vi "End Run.vi"(8 "abort":bool, 11 "RTTarget in":refnum<class "RTTarget.lvclass">) -> (3 "RTTarget out":refnum<class "RTTarget.lvclass">)   [LabVIEW 2020, in "NI_TargetHelper.lvlib" / "RTTarget.lvclass"]
uses:
  <vilib>/TargetSupport/NI_TargetHelper/RTTarget/RTTarget.lvclass
  <vilib>/TargetSupport/NI_TargetHelper/RTTarget/RTTarget.lvclass/RTTarget.ctl
  <vilib>/TargetSupport/NI_TargetHelper/Run Target VI.ctl
  <vilib>/TargetSupport/NI_TargetHelper/NI_TargetHelper.lvlib
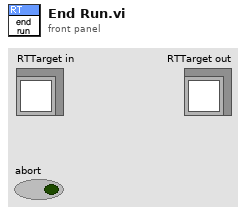
[diagram p1: front panel]
types:
  T1 = typedef "NI_TargetHelper.lvlib/Run Target VI.ctl" = refnum<vi>
  T2 = typedef "NI_TargetHelper.lvlib/Instance VIref.ctl" = refnum<vi>
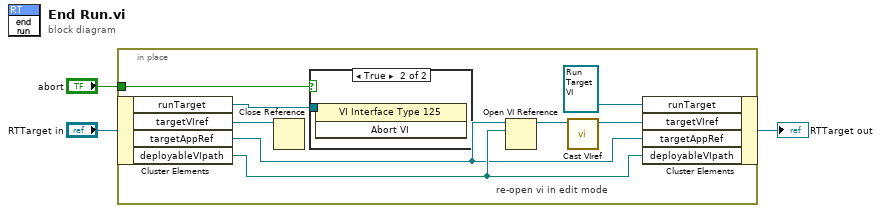
[diagram p0: block diagram]
diagram:
  n1 = in-place {
    in-place-border: "abort" -> [w10]
    # "re-open vi in edit mode"
    n2 = in-place-cluster #1("RTTarget in") -> ("runTarget"=w11:T1, "targetVIref"=w8:T2, "targetAppRef"=w4:refnum<vi>, "deployableVIpath"=w6:path)
    n3 = Close Reference(reference=w8) -> ()  [unwired: 1 in, 1 out]
    n4 = case shown="True" w10 {
      tunnel: w11 -> [_ w12]
      frame False {
      }
      frame True {
        n5 = invoke class="VI Interface Type 125" method="Abort VI"(reference=w12) -> ()  [unwired: 2 in, 3 out]
      }
    }
    n6 = Open VI Reference(application reference (local)=w4, vi path=w6) -> (vi reference=w7:refnum<vi>)  [unwired: 4 in, 1 out]
    n7 = call <vilib>:"Cast VIref.vi"("VI Refnum"=w7) -> ("instVIref"=w5:T2)  [unwired: 10 in]
    n8 = in-place-cluster #1("runTarget"=T1 refnum, "targetVIref"=w5, "targetAppRef"=w4, "deployableVIpath"=w6) -> (→"RTTarget out":refnum<class "RTTarget.lvclass">)
  }
